vi "Simple_Data_Monitor.vi"() -> ()   [LabVIEW 2016]
doc: "This example performs a serial port write and a serial port read. The parameters set for the serial port must match the parameters of the connected instrument or device. The VISA Configure Serial Port VI sets the configuration parameters. The front panel displays the controls used to configure the basic parameters, such as baud rate, data bits, and parity. The VI passes the VISA resource name to other VIs that perform operations on that VISA resource. The VISA Write function sends a command to the serial device and the VISA Read function returns data based on the command. The VISA Close function then closes the reference to the serial device. It is important to close the reference; otherwise, further communication through that port might not be possible."
uses:
  Program Files (x86)/National Instruments/LabVIEW 2016/examples/Instrument IO/Serial/support/Serial - Settings.ctl
  <vilib>/Instr/_visa.llb/VISA Configure Serial Port (Instr).vi
panel:
  in  "Tab Control":enum32{"Config", "Display"}(tab)
  in  "Serial Settings":T1={"baud rate"=9600, "data bits"=8, "parity"=enum."None", "stop bits"=10, "flow control"=0} {"flow control" items=["None"=0, "XON/XOFF"=1, "RTS/CTS"=2, "DTR/DSR"=4]; "stop bits" items=["1.0"=10, "1.5"=15, "2.0"=20]; "data bits" min=5 max=8 step=1; "baud rate" items=["75"=75, "110"=110, "134"=134, "150"=150, "300"=300, "600"=600, "1200"=1200, "1800"=1800, "2400"=2400, "4800"=4800, "7200"=7200, "9600"=9600, "14400"=14400, "19200"=19200, "28800"=28800, "38400"=38400, "56000"=56000, "57600"=57600, "115200"=115200, "128000"=128000, "230400"=230400]}
  in  "VISA resource name":refnum<visa-resource-name>="COM1"
  in  "termination char\n(0xA = '\\n' = LF)":u8=10 format="%.0x"
  out "Response":string
  out "wait":i32
  out "bytes read":u32
  out "array":dbl[](array[numeric])
  out "Waveform Chart":T2(graph)
  in  "stop":bool
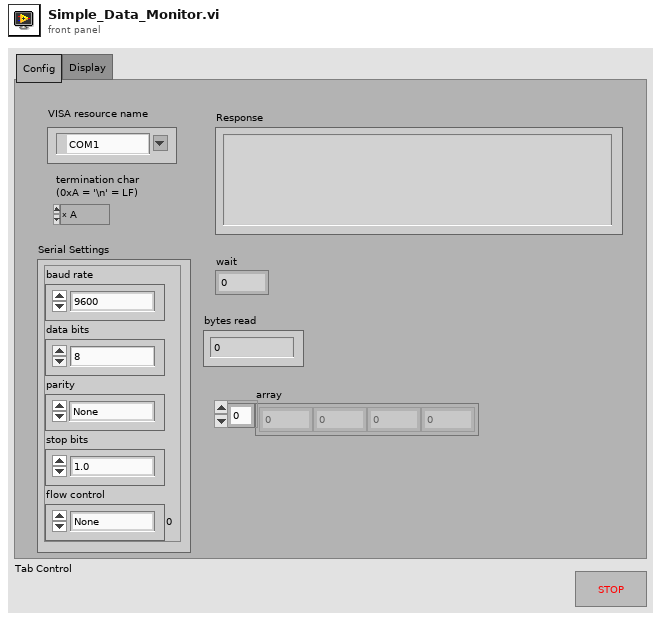
[diagram p1: front panel]
types:
  T1 = typedef "Serial - Settings.ctl" = cluster{"baud rate":u32, "data bits":u16, "parity":enum16{"None", "Odd", "Even", "Mark", "Space"}, "stop bits":u16, "flow control":u16}
  T2 = cluster{"array type (2D Dbl)[0]":dbl, "array type (2D Dbl)[1]":dbl, "array type (2D Dbl)[2]":dbl}
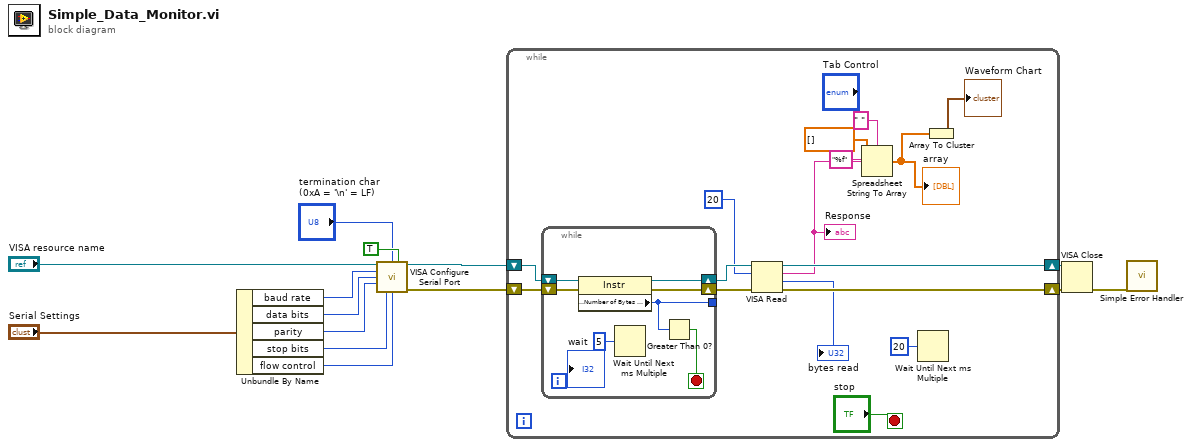
[diagram p0: block diagram]
diagram:
  n1 = Unbundle By Name("Serial Settings") -> ("baud rate"=w9:u32, "data bits"=w8:u16, "parity"=w7:enum16{"None", "Odd", "Even", "Mark", "Space"}, "stop bits"=w6:u16, "flow control"=w5:u16)
  n2 = call-poly "VISA Configure Serial Port"("VISA resource name"="VISA resource name", "termination char\n(0xA = '\\n' = LF)"="termination char\n(0xA = '\\n' = LF)", "Enable Termination\nChar (T)"=TRUE ("Enable Termination\nChar (T)"), "baud rate (9600)"=w9, "data bits (8)"=w8, "parity (0:none)"=w7, "stop bits (10: 1 bit)"=w6, "flow control (0:none)"=w5) -> ("VISA resource name out"=w2:refnum<visa-resource-name>, "error out"=w1:errorcluster)  [unwired: 2 in, 4 out]
  n3 = while {
    shift-right: [w29] -> w12
    shift-left: w2 -> [w26]
    shift-right: [w30] -> w13
    shift-left: w1 -> [w25]
    stop <- "stop" stop-if-true
    n4 = while {
      tunnel: [w33] -> _
      shift-right: [w38] -> w28
      shift-left: w26 -> [w36]
      shift-right: [w37] -> w27
      shift-left: w25 -> [w35]
      i -> [w31]
      stop <- w32 stop-if-true
      n5 = property class="Instr"(reference=w36, error in=w35) -> (reference out=w38:refnum<visa-resource-name>, error out=w37:errorcluster, "Serial Settings:Number of Bytes at Serial Port"=w33:u32)
      n6 = Wait Until Next ms Multiple(millisecond multiple=u32 5) -> ()  [unwired: 1 out]
      n7 = Greater Than 0?(x=w33) -> (x > 0?=w32:bool)
      "wait" <- w31
    }
    n8 = VISA Read(VISA resource name=w28, byte count=u32 20, error in (no error)=w27) -> (VISA resource name out=w29:refnum<visa-resource-name>, read buffer=w23:string, return count=→"bytes read":u32, error out=w30:errorcluster)
    "Response" <- w23
    n9 = Spreadsheet String To Array(delimiter (Tab)=" ", format string="%f", spreadsheet string=w23, array type (2D Dbl)=dbl[] []) -> (array=w19:dbl[])
    "array" <- w19
    n10 = Wait Until Next ms Multiple(millisecond multiple=u32 20) -> ()  [unwired: 1 out]
    n11 = Array To Cluster(array=w19) -> (cluster=→"Waveform Chart":T2)
  }
  n12 = VISA Close(VISA resource name=w12, error in (no error)=w13) -> (error out=w11:errorcluster)
  n13 = call <vilib>:"Simple Error Handler.vi"("error in (no error)"=w11) -> ()  [unwired: 1 in, 8 out]
